vi "Load SDF from Disk.vi"(8 "error in (no error)":errorcluster, 11 "refnum":T1) -> (0 "error out":errorcluster, 1 "Valid Path?":bool, 2 "SDF Path":path, 3 "refnum out":T1)   [LabVIEW 2016, in "System Mapping Tool.lvlib"]
uses:
  System Mapping Tool.lvlib
  <vilib>/Utility/config.llb/Config Data RefNum.ctl
  <vilib>/Utility/config.llb/NI_LVConfig.lvlib
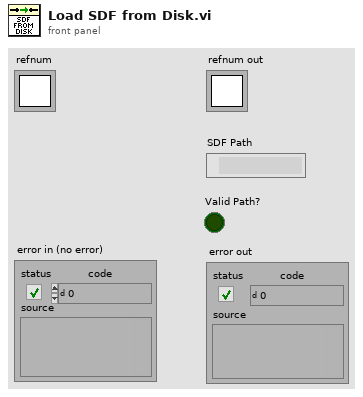
[diagram p1: front panel]
types:
  T1 = typedef "NI_LVConfig.lvlib/Config Data RefNum.ctl" = refnum<k1>
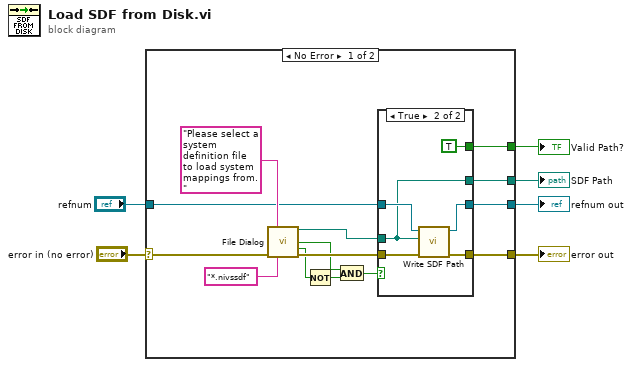
[diagram p0: block diagram]
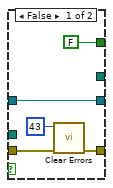
[diagram p2: hidden frame]
diagram:
  n1 = case shown="No Error" "error in (no error)" {
    selector: "error in (no error)" -> [w12 w33]
    tunnel: [w11 w33] -> w5
    tunnel: [w10 _] -> w4
    tunnel: [w9 _] -> w3
    tunnel: [w8 w32] -> w2
    tunnel: "refnum" -> [w7 w32]
    frame No Error {
      n2 = call "File Dialog"("prompt"="Please select a system definition file to load system mappings from.", "error in"=w12, "pattern (all files)"="*.nivssdf") -> ("selected path"=w17:path, "exists"=w16:bool, "cancelled"=w14:bool, "error out"=w18:errorcluster)  [unwired: 9 in]
      n3 = Not(x=w14) -> (.not. x?=w15:bool)
      n4 = And(x=w16, y=w15) -> (x .and. y?=w13:bool)
      n5 = case shown="True" w13 {
        tunnel: w18 -> [w24 w31]
        tunnel: [w22 w30] -> w11
        tunnel: w17 -> [_ w27]
        tunnel: w7 -> [w25 w29]
        tunnel: [w25 w28] -> w8
        tunnel: [_ w27] -> w9
        tunnel: [FALSE TRUE] -> w10
        frame False {
          n6 = call <vilib>:"Clear Errors.vi"("error in (no error)"=w24, "specific error code to clear (0: all)"=43) -> ("error out"=w22:errorcluster)  [unwired: 4 in, 1 out]
        }
        frame True {
          n7 = call "Write SDF Path.vi"("error in (no error)"=w31, "Path"=w27, "refnum"=w29) -> ("error out"=w30:errorcluster, "refnum out"=w28:T1)  [unwired: 7 in]
        }
      }
    }
    frame Error {
    }
  }
  "refnum out" <- w2
  "SDF Path" <- w3
  "Valid Path?" <- w4
  "error out" <- w5
